vi "SP Find and Convert Magnitude Limit.vi"(4 "Format":T7 caption="Display Format" items=["Log Mag", "Phase", "Expanded Phase", "Delay", "Smith", "Polar", "Lin Mag", "SWR", "Loss", "Real", "Imaginary"], 6 "Parameter":T3={"Stimulus Port"=1, "Response Port"=1} caption="Parameter String" {"Stimulus Port" min=1 step=1; "Response Port" min=1 step=1}, 7 "Limits":T2[](array[typedef]) {"Parameter"."Stimulus Port" min=1 step=1; "Parameter"."Response Port" min=1 step=1}) -> (0 "Limits":T2[](array[typedef]) {"Parameter"."Stimulus Port" min=1 step=1; "Parameter"."Response Port" min=1 step=1}, 3 "Limit Format":T1)   [LabVIEW 2011]
uses:
  TypeDefs/SP Limit.ctl
  TypeDefs/SP Parameter.ctl
  TypeDefs/SP Format.ctl
  TypeDefs/SP Limit Type.ctl
  TypeDefs/SP Limit Point.ctl
  Test Referential Limit.ctl
  TypeDefs/SP Display Format.ctl
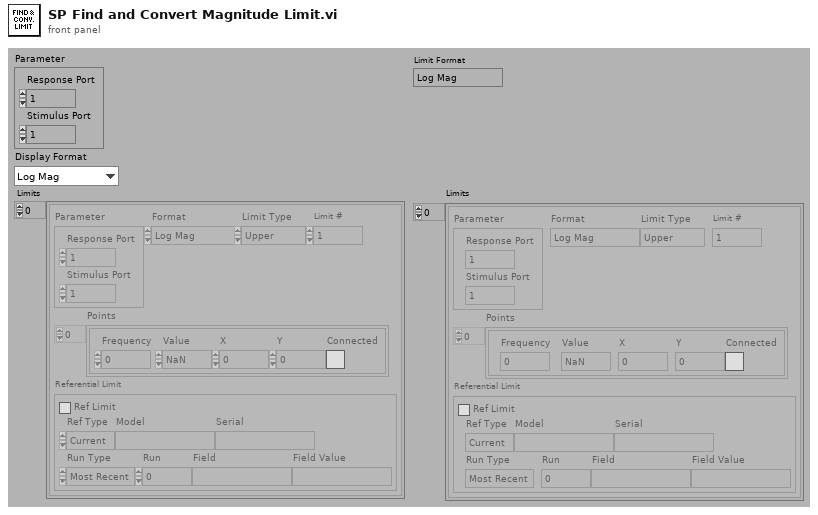
[diagram p1: front panel]
types:
  T1 = typedef "SP Format.ctl" = enum16{"Log Mag", "Lin Mag", "SWR", "Phase", "Expanded Phase", "Delay", "Insertion Loss", "Isolation", "Return Loss"}
  T2 = typedef "SP Limit.ctl" = cluster{"Parameter":T3, "Format":T1, "Limit Type":T4, "Points":T5[], "Referential Limit":T6, "Limit #":i8}
  T3 = typedef "SP Parameter.ctl" = cluster{"Stimulus Port":i8, "Response Port":i8}
  T4 = typedef "SP Limit Type.ctl" = enum16{"Upper", "Lower", "Delta", "Filter", "Referential"}
  T5 = typedef "SP Limit Point.ctl" = cluster{"Frequency":dbl, "Value":dbl, "X":dbl, "Y":dbl, "Connected":bool}
  T6 = typedef "Test Referential Limit.ctl" = cluster{"Ref Limit":bool, "Ref Type":enum16{"Current", "Specify"}, "Model":string, "Serial":string, "Run Type":enum16{"Most Recent", "Run #", "Match Field"}, "Run":i32, "Field":string, "Field Value":string}
  T7 = typedef "SP Display Format.ctl" = i32
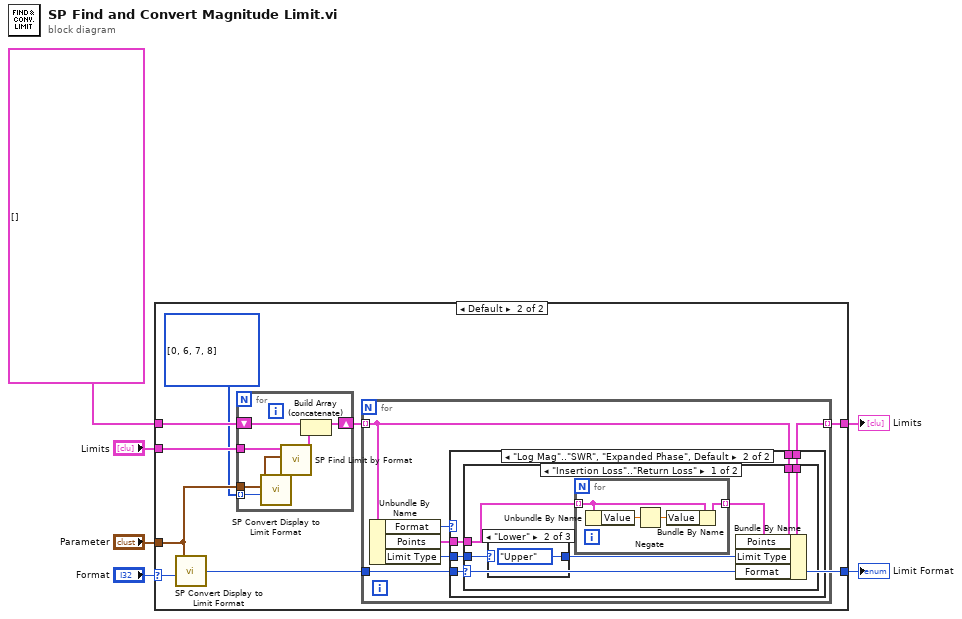
[diagram p0: block diagram]
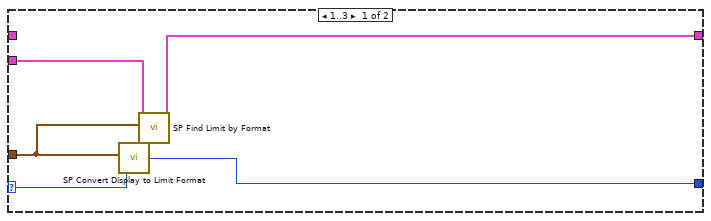
[diagram p2: hidden frame]
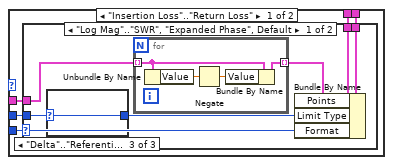
[diagram p3: hidden frame]
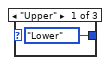
[diagram p4: hidden frame]
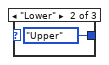
[diagram p5: hidden frame]
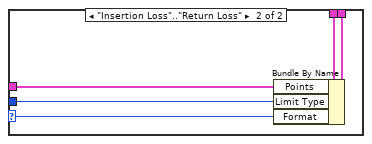
[diagram p6: hidden frame]
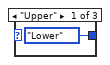
[diagram p7: hidden frame]
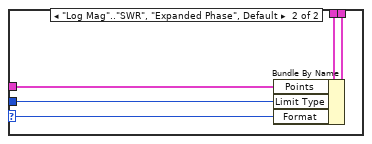
[diagram p9: hidden frame]
diagram:
  n1 = case shown="Default" "Format" {
    selector: "Format" -> [w10 w17]
    tunnel: "Limits" -> [w11 w19]
    tunnel: "Parameter" -> [w7 w18]
    tunnel: [w9 w13] -> w1
    tunnel: [w8 w16] -> w5
    tunnel: T2[] [] ("Limits") -> [_ w15]
    frame 1..3 {
      n2 = call "SP Convert Display to Limit Format.vi"("Display Format"=w10, "S Parameter"=w7) -> ("Limit Format"=w8:T1)  [unwired: 4 out]
      n3 = call "SP Find Limit by Format.vi"("Limit Format"=w8, "Parameter"=w7, "Limits"=w11) -> ("Limits"=w9:T2[])  [unwired: 8 out]
    }
    frame Default {
      w12 = T7[] [0, 6, 7, 8] items=["Log Mag", "Phase", "Expanded Phase", "Delay", "Smith", "Polar", "Lin Mag", "SWR", "Loss", "Real", "Imaginary"]
      n4 = call "SP Convert Display to Limit Format.vi"("Display Format"=w17, "S Parameter"=w18) -> ("Limit Format"=w16:T1)  [unwired: 4 out]
      n5 = for {
        tunnel: w19 -> [w80]
        tunnel: w18 -> [w74]
        tunnel: w12 -> [w79] mode=indexing
        shift-right: [w75] -> w14
        shift-left: w15 -> [w77]
        n6 = call "SP Convert Display to Limit Format.vi"("Display Format"=w79, "S Parameter"=w74) -> ("Limit Format"=w78:T1)  [unwired: 4 out]
        n7 = call "SP Find Limit by Format.vi"("Limit Format"=w78, "Parameter"=w74, "Limits"=w80) -> ("Limits"=w76:T2[])  [unwired: 8 out]
        n8 = Build Array (concatenate)(w77, w76) -> (w75:T2[])
      }
      n9 = for {
        tunnel: w14 -> [w20] mode=indexing
        tunnel: w16 -> [w23]
        tunnel: [w21] -> w13 mode=indexing
        n10 = Unbundle By Name(w20) -> ("Format"=w25:T1, "Points"=w24:T5[], "Limit Type"=w22:T4)
        n11 = case shown="\"Log Mag\"..\"SWR\", \"Expanded Phase\", Default" w25 {
          tunnel: w24 -> [w29 w52]
          tunnel: w23 -> [w30 w50]
          tunnel: w20 -> [w28 w54]
          tunnel: [w27 w53] -> w21
          tunnel: w22 -> [w26 w51]
          frame "Insertion Loss".."Return Loss" {
            n12 = case shown="\"Log Mag\"..\"SWR\", \"Expanded Phase\", Default" w30 {
              selector: w30 -> [w37 w47]
              tunnel: w29 -> [w32 w49]
              tunnel: w26 -> [w33 w48]
              tunnel: w28 -> [w36 w46]
              tunnel: [w35 w45] -> w27
              frame "Log Mag".."SWR", "Expanded Phase", Default {
                n13 = case shown="\"Delta\"..\"Referential\"" w33 {
                  selector: w33 -> [_ _ w44]
                  tunnel: [SP_Limit_Type."Lower" ("Limit Type") SP_Limit_Type."Upper" ("Limit Type") w44] -> w34
                  frame "Upper" {
                  }
                  frame "Lower" {
                  }
                  frame "Delta".."Referential" {
                  }
                }
                n14 = for {
                  tunnel: w32 -> [w41] mode=indexing
                  tunnel: [w40] -> w31 mode=indexing
                  n15 = Unbundle By Name(w41) -> ("Value"=w39:dbl)
                  n16 = Negate(x=w39) -> (-x=w38:dbl)
                  n17 = Bundle By Name(cluster=w41, "Value"=w38) -> (w40:T5)
                }
                n18 = Bundle By Name(cluster=w36, "Points"=w31, "Limit Type"=w34, "Format"=w37) -> (w35:T2)
              }
              frame "Insertion Loss".."Return Loss" {
                n19 = Bundle By Name(cluster=w46, "Points"=w49, "Limit Type"=w48, "Format"=w47) -> (w45:T2)
              }
            }
          }
          frame "Log Mag".."SWR", "Expanded Phase", Default {
            n20 = case shown="\"Insertion Loss\"..\"Return Loss\"" w50 {
              selector: w50 -> [w61 w71]
              tunnel: w52 -> [w56 w73]
              tunnel: w51 -> [w57 w72]
              tunnel: w54 -> [w60 w70]
              tunnel: [w59 w69] -> w53
              frame "Insertion Loss".."Return Loss" {
                n21 = case shown="\"Lower\"" w57 {
                  selector: w57 -> [_ _ w68]
                  tunnel: [SP_Limit_Type."Lower" ("Limit Type") SP_Limit_Type."Upper" ("Limit Type") w68] -> w58
                  frame "Upper" {
                  }
                  frame "Lower" {
                  }
                  frame "Delta".."Referential" {
                  }
                }
                n22 = for {
                  tunnel: w56 -> [w65] mode=indexing
                  tunnel: [w64] -> w55 mode=indexing
                  n23 = Unbundle By Name(w65) -> ("Value"=w63:dbl)
                  n24 = Negate(x=w63) -> (-x=w62:dbl)
                  n25 = Bundle By Name(cluster=w65, "Value"=w62) -> (w64:T5)
                }
                n26 = Bundle By Name(cluster=w60, "Points"=w55, "Limit Type"=w58, "Format"=w61) -> (w59:T2)
              }
              frame "Log Mag".."SWR", "Expanded Phase", Default {
                n27 = Bundle By Name(cluster=w70, "Points"=w73, "Limit Type"=w72, "Format"=w71) -> (w69:T2)
              }
            }
          }
        }
      }
    }
  }
  "Limits" <- w1
  "Limit Format" <- w5
